vi "Export Data.vi"(8 "error in (no error)":errorcluster, 11 "Data in":T10={"UI References"={"Stop Ref"=refnum, "Save Ref"=refnum, "Open Ref"=refnum, "Export Ref"=refnum, "Acquire Ref"=refnum, "Configure Ref"=refnum, "Graph Ref"=refnum, "Clear Ref"=refnum, "Analyze Ref"=refnum, "Status Ref"=refnum, "Snapshot Ref"=refnum}, "Graph Data"={"Data"=[], "Annotation List"=[], "Cursor List"=[], "Analysis Data"=[]}, "User Specified"={"Hardware Configuration"={"Signal Channel"="", "Response Channel"="", "Trigger Channel"="", "Number of acquisitions"=0.0}, "Analysis Configuration"={"Statistics"=TRUE}, "Signal Type"=enum."Single Chirp", "New Data Behavior"=enum."Replace", "Signal Configuration"={"Chirp Amplitude"=0.1, "I/O Limit"=10.0, "Sample Rate"=1000000.0, "Chirp Duration (s)"=10000000.0, "Upper Frequency"=0.0, "Lower Frequency"=0.0, "Windowing"=enum."None"}}}) -> (0 "error out":errorcluster)   [LabVIEW 2017]
doc: "Exports the currently displayed data and analysis to a tab separated text file suitable for loading in a spreadsheet application."
uses:
  controls/UI References.ctl
  controls/Graph Data.ctl
  <vilib>/Utility/miscctls.llb/LVAnnotationListTypeDef.ctl
  <vilib>/Utility/miscctls.llb/LVCursorListTypeDef.ctl
  controls/User Specified Data.ctl
  controls/HW Configuration.ctl
  controls/Analysis Configuration.ctl
  controls/New Data Behavior.ctl
  controls/Signal Configuration.ctl
  <vilib>/Waveform/WDTFileIO.llb/Export Waveforms To Spreadsheet File (1D).vi
panel:
  out "error out 2":errorcluster
  in  "error in (no error) 2":errorcluster
  # "(Scroll up to see large data cluster)"
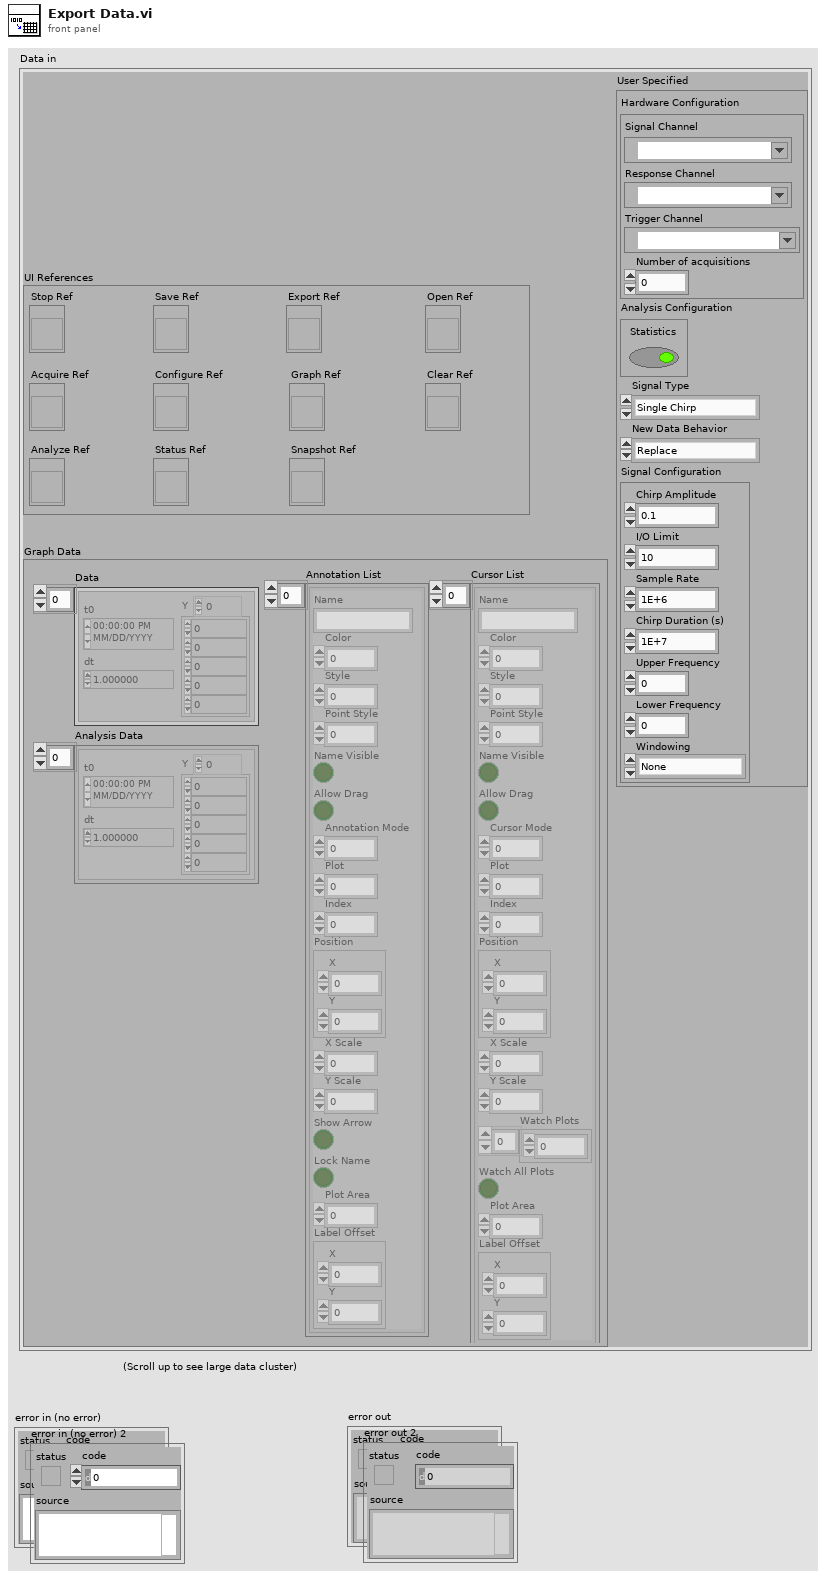
[diagram p1: front panel]
types:
  T1 = typedef "UI References.ctl" = cluster{"Stop Ref":refnum<vi>, "Save Ref":refnum<vi>, "Open Ref":refnum<vi>, "Export Ref":refnum<vi>, "Acquire Ref":refnum<vi>, "Configure Ref":refnum<vi>, "Graph Ref":refnum<vi>, "Clear Ref":refnum<vi>, "Analyze Ref":refnum<vi>, "Status Ref":refnum<vi>, "Snapshot Ref":refnum<vi>}
  T2 = typedef "Graph Data.ctl" = cluster{"Data":waveform(dbl)[], "Annotation List":T3, "Cursor List":T4, "Analysis Data":waveform(dbl)[]}
  T3 = typedef "LVAnnotationListTypeDef.ctl" = cluster{"Name":string, "Color":u32, "Style":u8, "Point Style":u8, "Name Visible":bool, "Allow Drag":bool, "Annotation Mode":u32, "Plot":i32, "Index":i32, "Position":cluster{"X":dbl, "Y":dbl}, "X Scale":u32, "Y Scale":u32, "Show Arrow":bool, "Lock Name":bool, "Plot Area":i32, "Label Offset":cluster{"X":dbl, "Y":dbl}}[]
  T4 = typedef "LVCursorListTypeDef.ctl" = cluster{"Name":string, "Color":u32, "Style":u8, "Point Style":u8, "Name Visible":bool, "Allow Drag":bool, "Cursor Mode":u32, "Plot":i32, "Index":i32, "Position":cluster{"X":dbl, "Y":dbl}, "X Scale":u32, "Y Scale":u32, "Watch Plots":i32[], "Watch All Plots":bool, "Plot Area":i32, "Label Offset":cluster{"X":dbl, "Y":dbl}}[]
  T5 = typedef "User Specified Data.ctl" = cluster{"Hardware Configuration":T6, "Analysis Configuration":T7, "Signal Type":enum16{"Single Chirp", "From Excel"}, "New Data Behavior":T8, "Signal Configuration":T9}
  T6 = typedef "HW Configuration.ctl" = cluster{"Signal Channel":tag, "Response Channel":tag, "Trigger Channel":tag, "Number of acquisitions":dbl}
  T7 = typedef "Analysis Configuration.ctl" = cluster{"Statistics":bool}
  T8 = typedef "New Data Behavior.ctl" = enum16{"Replace", "Overlay", "Append"}
  T9 = typedef "Signal Configuration.ctl" = cluster{"Chirp Amplitude":dbl, "I/O Limit":dbl, "Sample Rate":dbl, "Chirp Duration (s)":dbl, "Upper Frequency":dbl, "Lower Frequency":dbl, "Windowing":enum16{"None", "Exponential", "Flat top", "Hamming", "Hanning", "Kaiser-Bessel", "Rectangular"}}
  T10 = cluster{"UI References":T1, "Graph Data":T2, "User Specified":T5}
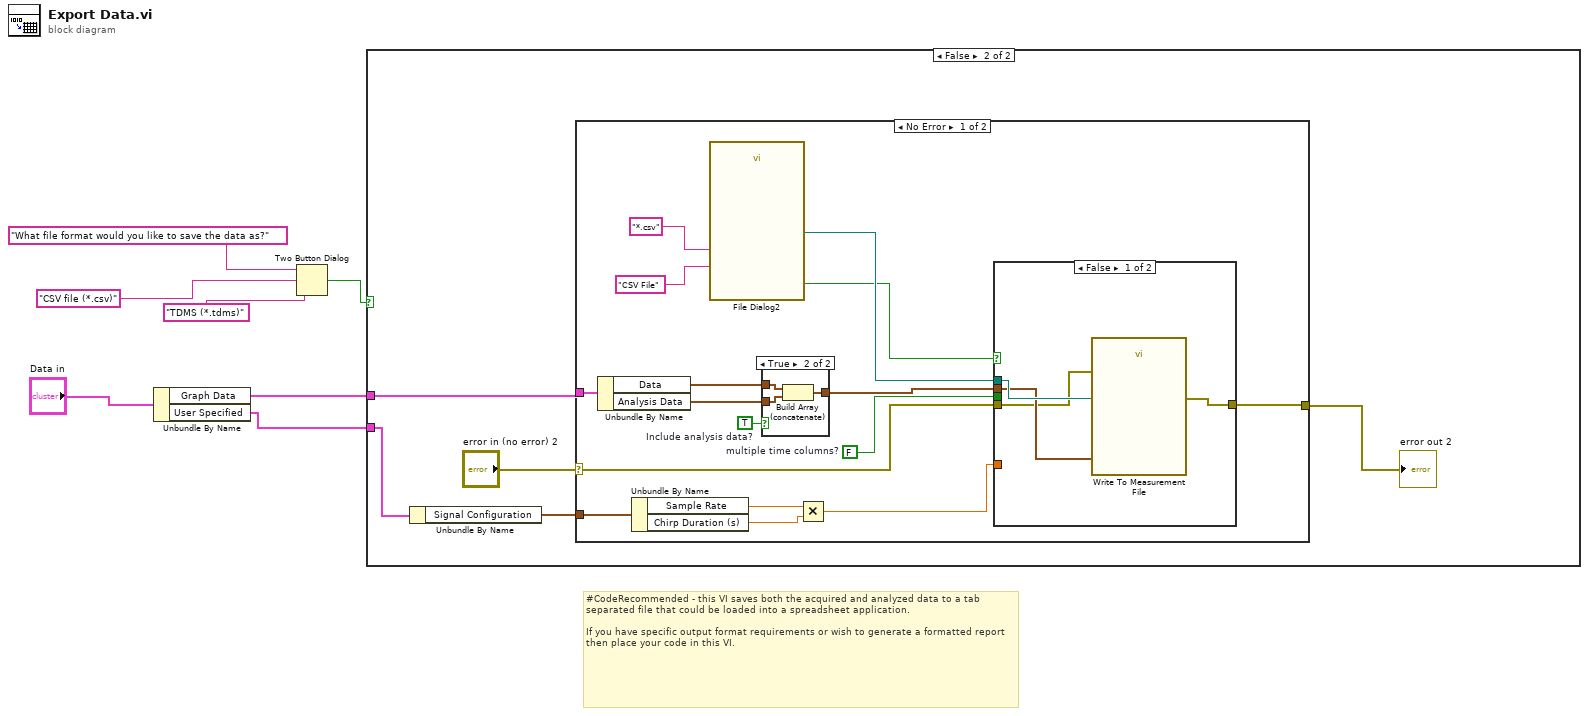
[diagram p0: block diagram]
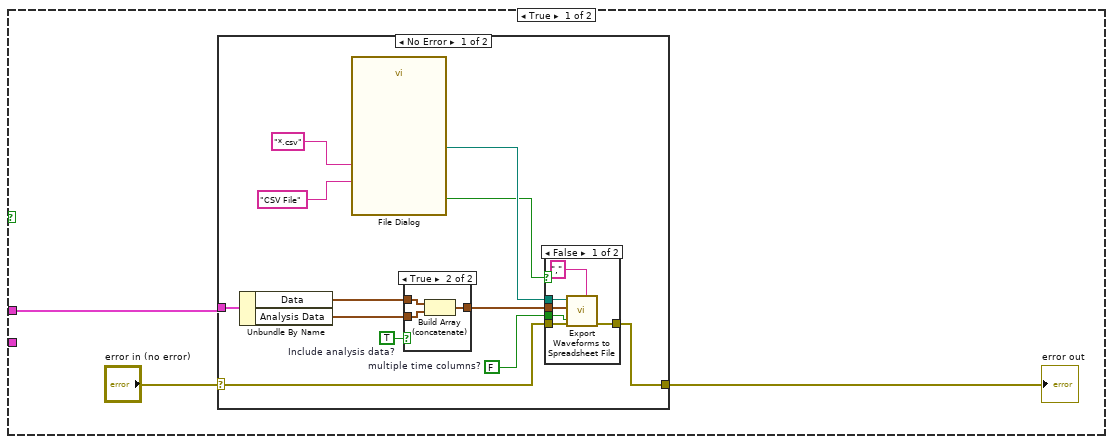
[diagram p2: hidden frame]
diagram:
  # "#CodeRecommended - this VI saves both the acquired and analyzed data to a tab separated file that could be loaded into a spreadsheet application.\n\nIf you have specific output format requirements or wish to generate a formatted report then place your code in this VI."
  n1 = Unbundle By Name("Data in") -> ("Graph Data"=w2:T2, "User Specified"=w1:T5)
  n2 = Two Button Dialog(message="What file format would you like to save the data as?", 1:"TDMS (*.tdms)" ("F button name (\"Cancel\")"), 2:"CSV file (*.csv)" ("T button name (\"OK\")")) -> (T button?=w4:bool)
  n3 = case shown="False" w4 {
    tunnel: w2 -> [w8 w37]
    tunnel: w1 -> [_ w36]
    frame True {
      n4 = case shown="No Error" "error in (no error)" {
        selector: "error in (no error)" -> [w20 w34]
        tunnel: w8 -> [w22 _]
        tunnel: [w19 w34] -> w9
        frame No Error {
          w15 = TRUE  # Include analysis data?
          w21 = FALSE  # multiple time columns?
          n5 = Unbundle By Name(w22) -> ("Data"=w18:waveform(dbl)[], "Analysis Data"=w17:waveform(dbl)[])
          n6 = call "File Dialog"("pattern (all files)"="*.csv", "pattern label"="CSV File" ("Text File")) -> ("selected path"=w14:path, "cancelled"=w11:bool)  [unwired: 10 in, 2 out]
          n7 = case shown="True" w15 {
            tunnel: w18 -> [w30 w33]
            tunnel: w17 -> [_ w32]
            tunnel: [w30 w31] -> w16
            frame False {
            }
            frame True {
              n8 = Build Array (concatenate)(w33, w32) -> (w31:waveform(dbl)[])
            }
          }
          n9 = case shown="False" w11 {
            tunnel: w21 -> [w28 _]
            tunnel: w20 -> [w27 w29]
            tunnel: [w26 w29] -> w19
            tunnel: w16 -> [w25 _]
            tunnel: w14 -> [w24 _]
            frame False {
              n10 = call-poly <vilib>:"Export Waveforms to Spreadsheet File.vi"("delimiter (Tab)"=",", "append to file? (new file:F)"=w28, "error in (no error)"=w27, "waveforms"=w25, "file path (dialog if empty)"=w24) -> ("error out"=w26:errorcluster)  [unwired: 5 in, 1 out]
            }
            frame True {
            }
          }
        }
        frame Error {
        }
      }
      "error out" <- w9
    }
    frame False {
      n11 = Unbundle By Name(w36) -> ("Signal Configuration"=w35:T9)
      n12 = case shown="No Error" "error in (no error) 2" {
        selector: "error in (no error) 2" -> [w53 w65]
        tunnel: w37 -> [w55 _]
        tunnel: [w52 w65] -> w38
        tunnel: w35 -> [w43 _]
        frame No Error {
          w48 = TRUE  # Include analysis data?
          w54 = FALSE  # multiple time columns?
          n13 = Unbundle By Name(w55) -> ("Data"=w51:waveform(dbl)[], "Analysis Data"=w50:waveform(dbl)[])
          n14 = Unbundle By Name(w43) -> ("Sample Rate"=w42:dbl, "Chirp Duration (s)"=w41:dbl)
          n15 = call "File Dialog2"("pattern (all files)"="*.csv", "pattern label"="CSV File" ("Text File")) -> ("selected path"=w47:path, "cancelled"=w44:bool)  [unwired: 10 in, 2 out]
          n16 = case shown="True" w48 {
            tunnel: w51 -> [w61 w64]
            tunnel: w50 -> [_ w63]
            tunnel: [w61 w62] -> w49
            frame False {
            }
            frame True {
              n17 = Build Array (concatenate)(w64, w63) -> (w62:waveform(dbl)[])
            }
          }
          n18 = Multiply(x=w42, y=w41) -> (x*y=w40:dbl)
          n19 = case shown="False" w44 {
            tunnel: w54 -> [_ _]
            tunnel: w53 -> [w57 w60]
            tunnel: [w56 w60] -> w52
            tunnel: w49 -> [w58 _]
            tunnel: w47 -> [w59 _]
            tunnel: w40 -> [_ _]
            frame False {
              n20 = call "Write To Measurement File"("Signals"=w58, "error in (no error)"=w57, "Filename"=w59) -> ("error out"=w56:errorcluster)  [unwired: 14 in, 2 out]
            }
            frame True {
            }
          }
        }
        frame Error {
        }
      }
      "error out 2" <- w38
    }
  }
